vi "Imaging button boolean text.vi"(9 "Ctrl refs cluster":T1, 10 "Imaging button boolean text":string, 11 "Acquisition button boolean text":string) -> ()   [LabVIEW 2017]
uses:
  Typedefs/ROI entry screen ctrl refs cluster.ctl
  Typedefs/Line draw mode.ctl
  Typedefs/ROI move mode.ctl
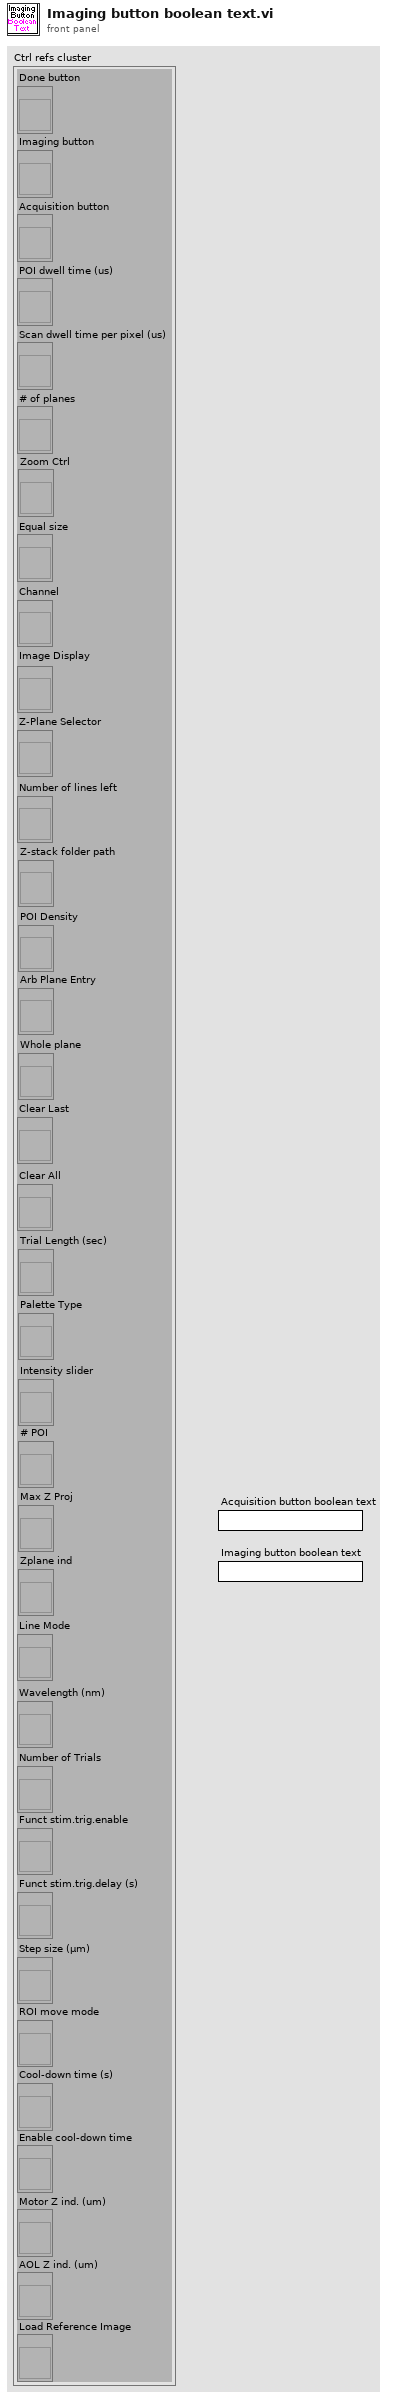
[diagram p1: front panel]
types:
  T1 = typedef "ROI entry screen ctrl refs cluster.ctl" = cluster{"Done button":refnum<vi>, "Imaging button":refnum<vi>, "Acquisition button":refnum<vi>, "POI dwell time (us)":refnum<vi>, "Scan dwell time per pixel (us)":refnum<vi>, "# of planes":refnum<vi>, "Zoom Ctrl":refnum<vi>, "Equal size":refnum<vi>, "Channel":refnum<vi>, "Image Display":refnum<vi>, "Z-Plane Selector":refnum<vi>, "Number of lines left":refnum<vi>, "Z-stack folder path":refnum<vi>, "POI Density":refnum<vi>, "Arb Plane Entry":refnum<vi>, "Whole plane":refnum<vi>, "Clear Last":refnum<vi>, "Clear All":refnum<vi>, "Trial Length (sec)":refnum<vi>, "Palette Type":refnum<vi>, "Intensity slider":refnum<vi>, "# POI":refnum<vi>, "Max Z Proj":refnum<vi>, "Zplane ind":refnum<vi>, "Wavelength (nm)":refnum<vi>, "Number of Trials":refnum<vi>, "Funct stim.trig.enable":refnum<vi>, "Funct stim.trig.delay (s)":refnum<vi>, "Line Mode":refnum<vi>, "Step size (µm)":refnum<vi>, "ROI move mode":refnum<vi>, "Cool-down time (s)":refnum<vi>, "Enable cool-down time":refnum<vi>, "Motor Z ind. (um)":refnum<vi>, "AOL Z ind. (um)":refnum<vi>, "Load Reference Image":refnum<vi>}
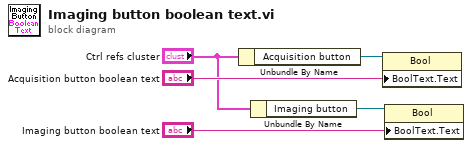
[diagram p0: block diagram]
diagram:
  n1 = Unbundle By Name("Ctrl refs cluster") -> ("Acquisition button"=w4:refnum<vi>)
  n2 = Unbundle By Name("Ctrl refs cluster") -> ("Imaging button"=w3:refnum<vi>)
  n3 = property on="Property Node" class="Bool"(reference=w4, "BoolText.Text"="Acquisition button boolean text") -> ()  [unwired: 1 in, 2 out]
  n4 = property on="Property Node" class="Bool"(reference=w3, "BoolText.Text"="Imaging button boolean text") -> ()  [unwired: 1 in, 2 out]
